vi "build help message.vi"(1 "Options":T1[](array[typedef])) -> (0 "help":string)   [LabVIEW 2024]
uses:
  <vilib>/addons/g-sugar/g-sugar.lvlib
  <vilib>/Wiresmith Technology/G CLI/Argument Parser/Option Class/Argument Type.ctl
  <vilib>/Wiresmith Technology/G CLI/Argument Parser/Option Class/Option.lvclass
  <vilib>/Wiresmith Technology/G CLI/Argument Parser/Option Class/Option Configuration.ctl
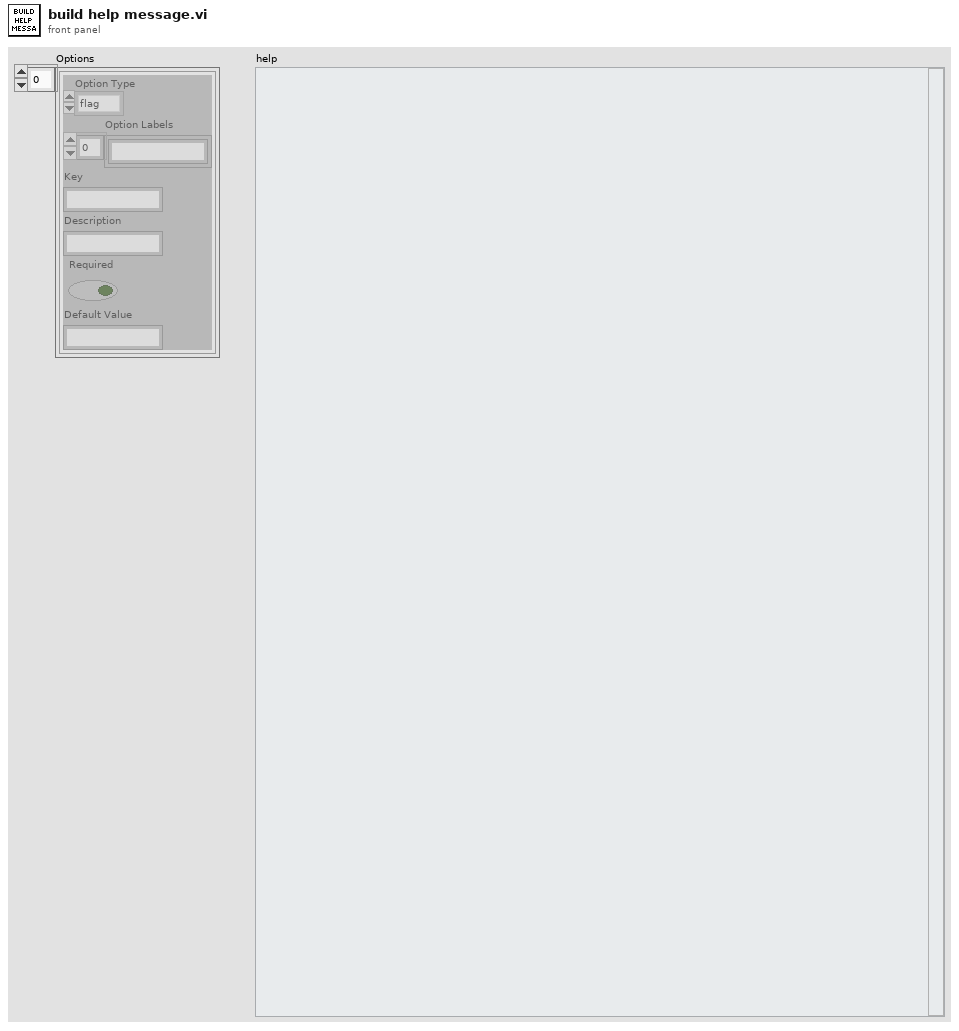
[diagram p1: front panel]
types:
  T1 = typedef "Option Parser.lvlib/Option.lvclass/Option Configuration.ctl" = cluster{"Option Type":T2, "Option Labels":string[], "Key":string, "Description":string, "Required":bool, "Default Value":string}
  T2 = typedef "Option Parser.lvlib/Option.lvclass/Argument Type.ctl" = enum16{"flag", "value"}
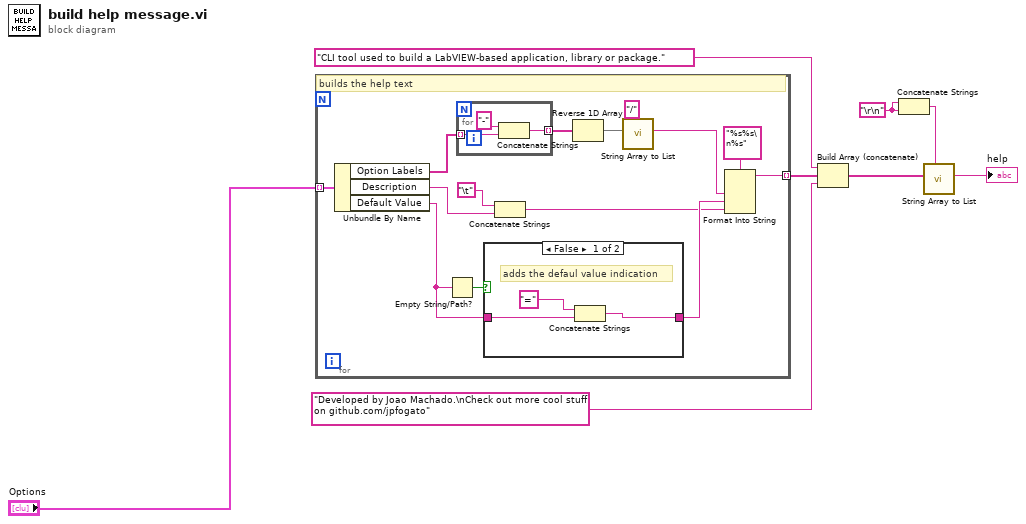
[diagram p0: block diagram]
diagram:
  w5 = "\r\n"
  n1 = for {
    tunnel: "Options" -> [w22] mode=indexing
    tunnel: [w15] -> w2 mode=indexing
    # "builds the help text"
    n2 = Unbundle By Name(w22) -> ("Option Labels"=w14:string[], "Description"=w12:string, "Default Value"=w9:string)
    n3 = Empty String/Path?(string/path=w9) -> (empty?=w17:bool)
    n4 = for {
      tunnel: w14 -> [w25] mode=indexing
      tunnel: [w24] -> w13 mode=indexing
      n5 = Concatenate Strings("-" ("string"), w25) -> (w24:string)
    }
    n6 = case shown="False" w17 {
      tunnel: w9 -> [w28 w29]
      tunnel: [w26 w29] -> w16
      frame False {
        # "adds the defaul value indication"
        n7 = Concatenate Strings("=" ("string"), w28) -> (w26:string)
      }
      frame True {
        # "do nothing if not populated"
      }
    }
    n8 = Concatenate Strings("\t", w12) -> (w11:string)
    n9 = Reverse 1D Array(array=w13) -> (reversed array=w20:string[])
    n10 = call <vilib>:"String Array to List.vi"("delimiter (, )"="/", "string array"=w20) -> ("delimited string"=w19:string)  [unwired: 9 in]
    n11 = Format Into String(format string="%s%s\n%s", w19, w16, w11) -> (resulting string=w15:string)  [unwired: 2 in, 1 out]
  }
  n12 = Build Array (concatenate)("CLI tool used to build a LabVIEW-based application, library or package." ("delimiter (, )"), w2, "Developed by Joao Machado.\nCheck out more cool stuff on github.com/jpfogato" ("delimiter (, )")) -> (w6:string[])
  n13 = Concatenate Strings(w5, w5) -> (w4:string)
  n14 = call <vilib>:"String Array to List.vi"("delimiter (, )"=w4, "string array"=w6) -> ("delimited string"=→"help":string)  [unwired: 9 in]
